vi "BASE.Device.Connect.vi"(8 "error in (no error)":errorcluster, 10 "Timeout (5000 ms)":i32, 11 "Device.Simulation in":refnum<class "Device.Simulation.lvclass">) -> (0 "error out":errorcluster, 2 "Connected?":bool, 3 "Device.Simulation out":refnum<class "Device.Simulation.lvclass">)   [LabVIEW 2019, in "Device.Simulation.lvlib" / "Device.Simulation.lvclass"]
uses:
  Device.Simulation.lvclass
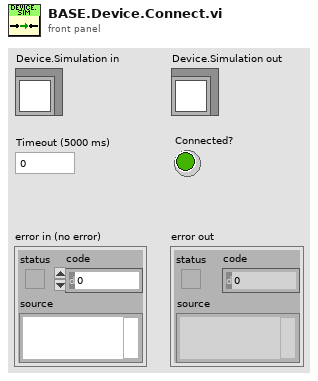
[diagram p1: front panel]
types:
  T1 = typedef "Device.Simulation.lvlib/Device.Simulation.lvclass/config--cluster.ctl" = cluster{"Name":string, "Time to Connect (ms)":u32, "Time to Check Connection (ms)":u32, "Time to Disconnect (ms)":u32, "Time to Read State (ms)":u32}
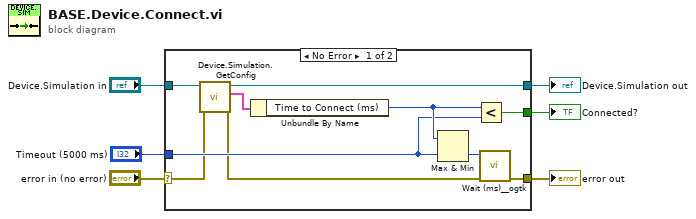
[diagram p0: block diagram]
diagram:
  n1 = case shown="No Error" "error in (no error)" {
    selector: "error in (no error)" -> [w10 w18]
    tunnel: [w16 w18] -> w5
    tunnel: "Device.Simulation in" -> [w11 w17]
    tunnel: [w8 w17] -> w3
    tunnel: "Timeout (5000 ms)" -> [w13 _]
    tunnel: [w12 _] -> w1
    frame No Error {
      n2 = call "Device.Simulation.GetConfig.vi"("error in (no error)"=w10, "Device.Simulation in"=w11) -> ("error out"=w9:errorcluster, "config"=w7:T1, "Device.Simulation out"=w8:refnum<class "Device.Simulation.lvclass">)  [unwired: 7 in]
      n3 = Unbundle By Name(w7) -> ("Time to Connect (ms)"=w14:u32)
      n4 = Max & Min(x=w14, y=w13) -> (min(x,y)=w15:u32)  [unwired: 1 out]
      n5 = Less?(x=w14, y=w13) -> (x < y?=w12:bool)
      n6 = call <userlib>:"Wait (ms)__ogtk.vi"("error in (no error)"=w9, "milliseconds to wait"=w15) -> ("error out"=w16:errorcluster)  [unwired: 8 in, 1 out]
    }
    frame Error {
    }
  }
  "error out" <- w5
  "Device.Simulation out" <- w3
  "Connected?" <- w1
